vi "Read Display - Low Limit.vi"(8 "error in (no error)":errorcluster, 11 "NT Scalar (Numeric) in":refnum<class "NT Scalar (Numeric).lvclass">) -> (0 "error out":errorcluster, 2 "low limit":dbl, 3 "NT Scalar (Numeric) out":refnum<class "NT Scalar (Numeric).lvclass">)   [LabVIEW 2020, in "PV Access.lvlib" / "PV Data.lvlib" / "NT Scalar (Numeric).lvclass"]
uses:
  NT Scalar (Numeric).lvclass
  75c87a2a-13fc-4ee2-8384-e32322e3cb61.vi
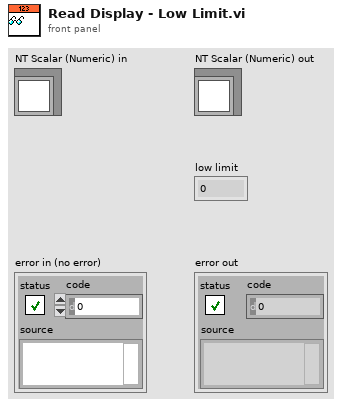
[diagram p1: front panel]
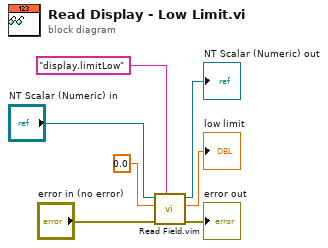
[diagram p0: block diagram]
diagram:
  n1 = call "Read Field.vim"("field"="display.limitLow", "error in"="error in (no error)", "default value"=0.0, "Base Interface in"="NT Scalar (Numeric) in") -> ("error out"=→"error out":errorcluster, "value"=→"low limit":dbl, "Base Interface out"=→"NT Scalar (Numeric) out":refnum<class "NT Scalar (Numeric).lvclass">)  [unwired: 5 in]
